vi "BER_Curve.vi"() -> ()   [LabVIEW 2013]
panel:
  out "Waveform Graph":dbl[](graph)
  in  "Samples":i32=16
  in  "Sample Step":dbl=0.3
  in  "Message Bits":i32=2000
  in  "Synchronization Sequence":i32=20
  in  "Zero Pad":i32=16
  out "Error Out":errorcluster
  in  "M-PSK":i32=4
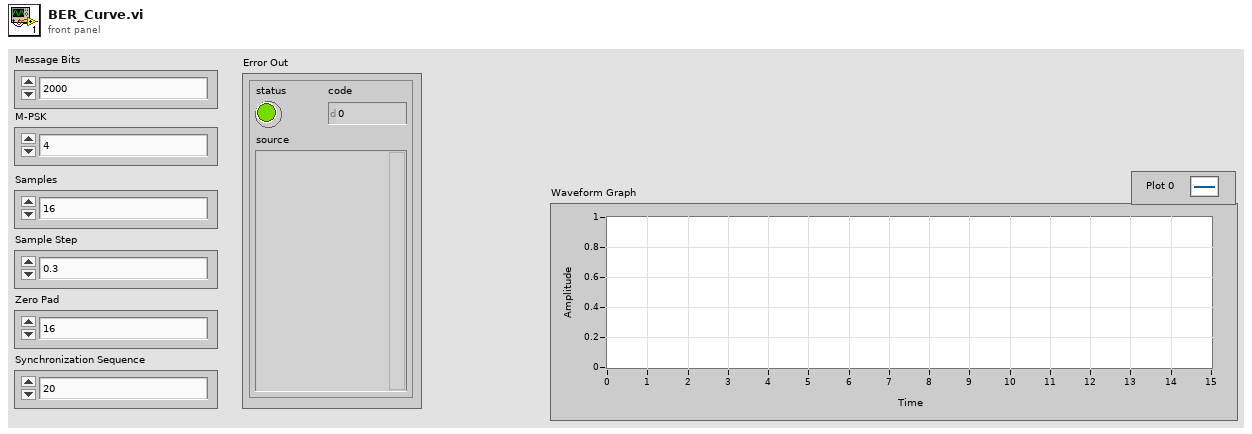
[diagram p1: front panel]
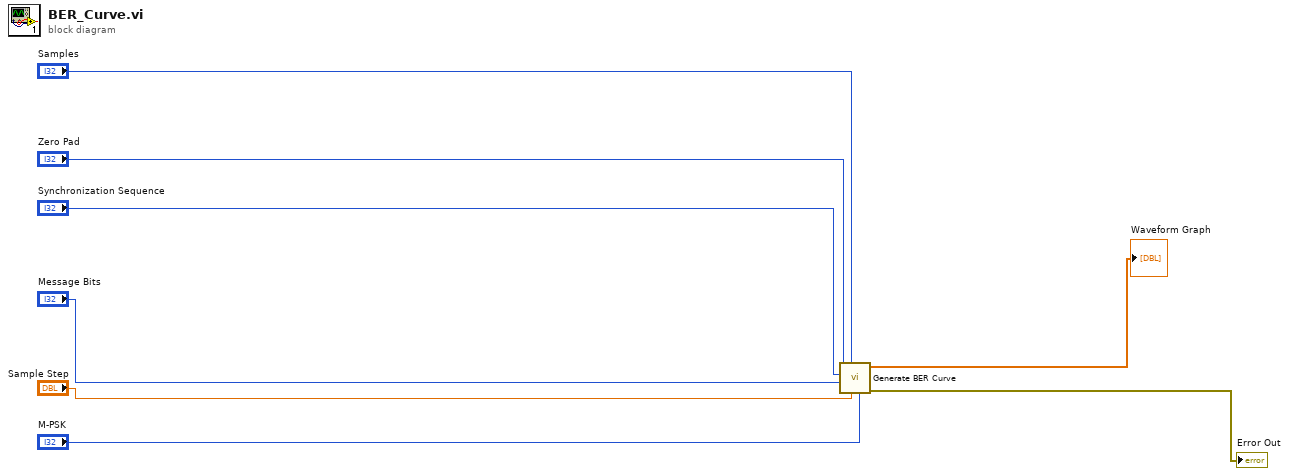
[diagram p0: block diagram]
diagram:
  n1 = call "Generate BER Curve.vi"("M-PSK"="M-PSK", "Sample Step"="Sample Step", "Samples"="Samples", "Message Bits"="Message Bits", "Synchronization Sequence"="Synchronization Sequence", "Zero Pad"="Zero Pad") -> ("error out"=→"Error Out":errorcluster, "BER Curve"=→"Waveform Graph":dbl[])  [unwired: 4 in]
